vi "Simple Network Streams - Target.vi"() -> ()   [LabVIEW 2015]
doc: "Demonstrates how to use Network Streams to pass data and commands between two running VIs. This VI passes data to the host VI, based on the frequency specified by the host VI."
uses:
  Control 1.ctl
  <vilib>/Platform/TimedLoop/XDataNode/timing_clust.ctl
  <vilib>/Platform/TimedLoop/XDataNode/nitl_modes.ctl
  <vilib>/Platform/TimedLoop/XDataNode/wakeup.ctl
  <vilib>/platform/TimedLoop/XDataNode/XDataNode.xnode
  <vilib>/ErrorRing/Error Ring.xnode
  <vilib>/Platform/TimedLoop/XDataNode/XDNodeRunTimeDep.lvlib
panel:
  out "Time":u32
  out "Counter":i32
  out "output cluster":T1
  in  "Stop":bool
  # "Overview: Demonstrates how to use Network Streams to pass data and commands between two running VIs.\nRequirements: Windows\nInstructions:\n1. Run this VI.\n2. Open Simple Network Streams - Host.vi and follow the instructions on its front panel."
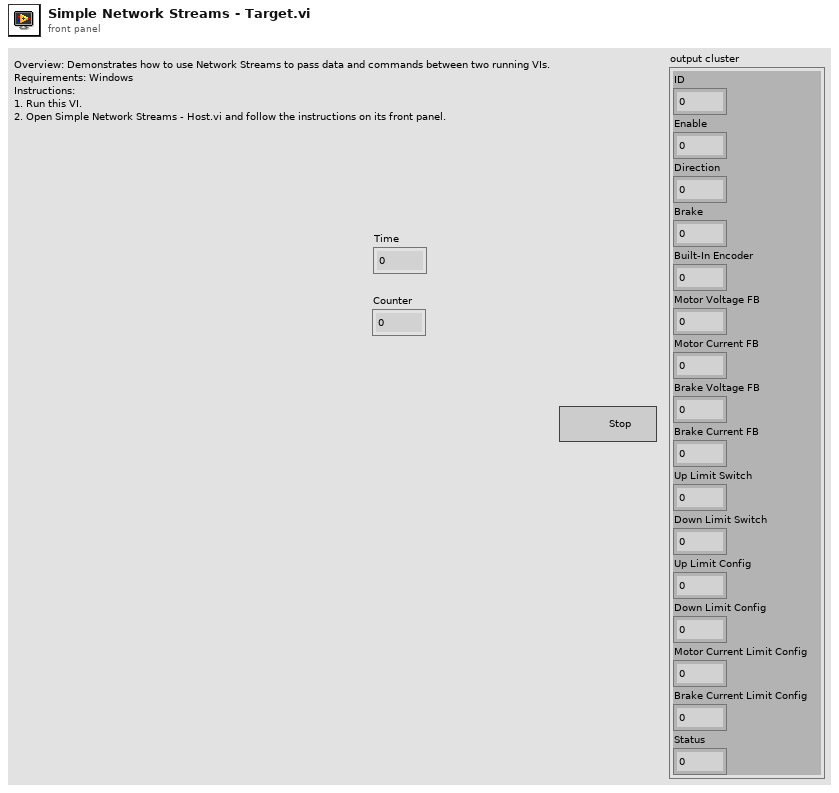
[diagram p1: front panel]
types:
  T1 = typedef "Control 1.ctl" = cluster{"ID":dbl, "Enable":dbl, "Direction":dbl, "Brake":dbl, "Built-In Encoder":dbl, "Motor Voltage FB":dbl, "Motor Current FB":dbl, "Brake Voltage FB":dbl, "Brake Current FB":dbl, "Up Limit Switch":dbl, "Down Limit Switch":dbl, "Up Limit Config":dbl, "Down Limit Config":dbl, "Motor Current Limit Config":dbl, "Brake Current Limit Config":dbl, "Status":dbl}
  T2 = cluster{"ID":dbl, "Enable":dbl, "Direction":dbl, "Brake":dbl, "Built-In Encoder":dbl, "Motor Voltage FB":dbl, "Motor Current FB":dbl, "Brake Voltage FB":dbl, "Brake Current FB":dbl, "Up Limit Switch":dbl, "Down Limit Switch":dbl, "Up Limit Config":dbl, "Down Limit Config":dbl, "Motor Current Limit Config":dbl, "Brake Current Limit Config":dbl, "Status":dbl}
  T3 = typedef "XDNodeRunTimeDep.lvlib/timing_clust.ctl" = cluster{"Expected End [f-1]":u64, "Actual End [f-1]":u64, "Finished Late? [f-1]":bool, "Expected End [i-1]":u64, "Actual End [i-1]":u64, "Finished Late? [i-1]":bool, "Expected Start [i]":u64, "Actual Start [i]":u64, "Expected Start [f]":u64, "Actual Start [f]":u64, "Source Name":string, "Structure Name":string, "Period":i64, "Deadline":i64, "Offset":i64, "Start":i64, "Priority":i32, "Timeout":i32, "Mode":T4, "Wakeup Reason":T5, "Error":errorcluster, "Source Type":string, "Secondary Source Type":string, "Global End Time":u64, "Global Start Time":u64, "Frame Duration":u64, "Iteration Duration":u64, "Assigned CPU":i32, "I/O Scan Engine Mode":u32}
  T4 = typedef "XDNodeRunTimeDep.lvlib/nitl_modes.ctl" = enum32{"No Change", "Process missed periods, maintain original phase", "Discard missed periods, maintain original phase", "Process missed periods, ignore original phase", "Discard missed periods, ignore original phase"}
  T5 = typedef "XDNodeRunTimeDep.lvlib/wakeup.ctl" = enum32{"Normal", "Aborted", "Asynchronous wakeup", "Timing source error", "Timed loop error", "Timeout"}
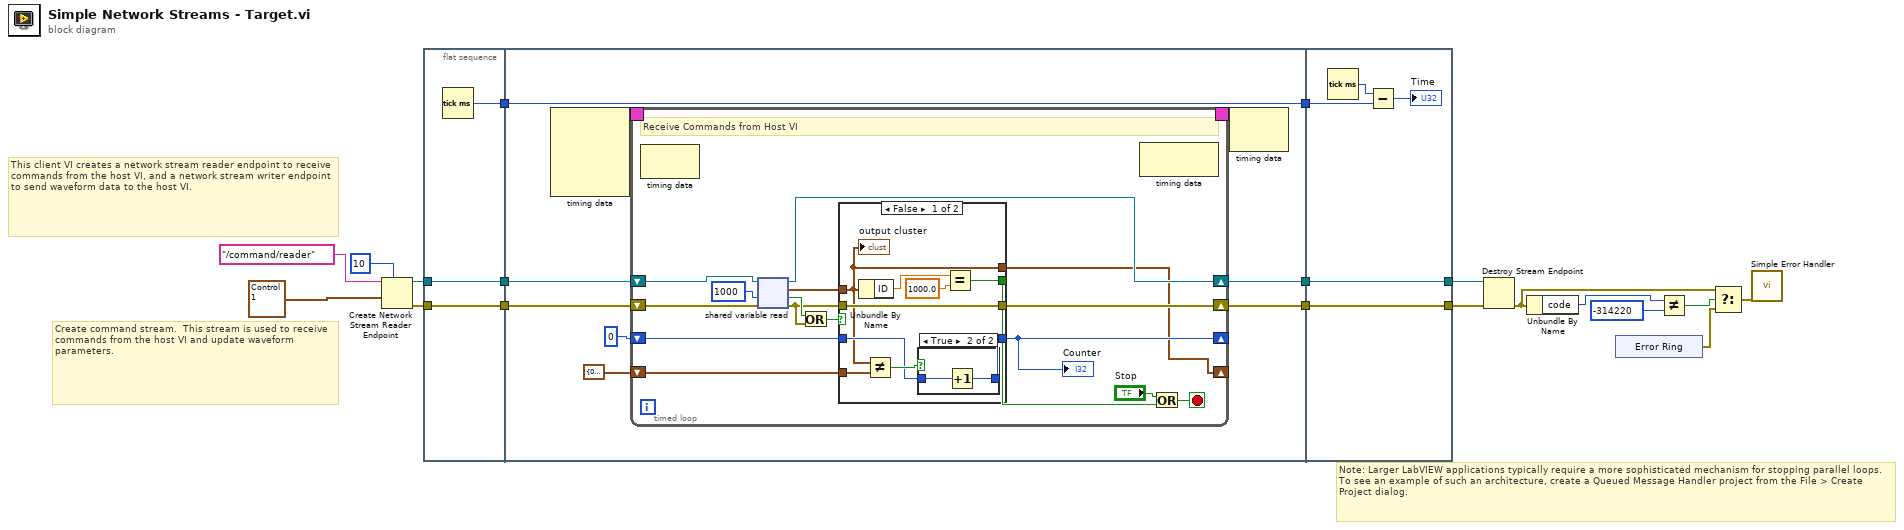
[diagram p0: block diagram]
diagram:
  # "This client VI creates a network stream reader endpoint to receive commands from the host VI, and a network stream writer endpoint to send waveform data to the host VI."
  # "Note: Larger LabVIEW applications typically require a more sophisticated mechanism for stopping parallel loops. To see an example of such an architecture, create a Queued Message Handler project from the File > Create Project dialog."
  # "Create command stream.  This stream is used to receive commands from the host VI and update waveform parameters."
  n1 = Create Network Stream Reader Endpoint(7:10 ("reader buffer size"), 9:T1 {"ID"=0.0, "Enable"=0.0, "Direction"=0.0, "Brake"=0.0, "Built-In Encoder"=0.0, "Motor Voltage FB"=0.0, "Motor Current FB"=0.0, "Brake Voltage FB"=0.0, "Brake Current FB"=0.0, "Up Limit Switch"=0.0, "Down Limit Switch"=0.0, "Up Limit Config"=0.0, "Down Limit Config"=0.0, "Motor Current Limit Config"=0.0, "Brake Current Limit Config"=0.0, "Status"=0.0} ("output cluster"), 11:"/command/reader" ("reader url")) -> (0:w17:errorcluster, 3:w18:refnum<k21>)  [unwired: 4 in]
  n2 = flat-sequence {
    tunnel: w17 -> [w21]
    tunnel: w18 -> [w22]
    tunnel: [w22] -> w6
    tunnel: [w21] -> w5
    tunnel: [w20] -> w1
    tunnel: w6 -> [w31]
    tunnel: w5 -> [w30]
    tunnel: [w29] -> w4
    tunnel: [w28] -> w3
    tunnel: [w26] -> w2
    tunnel: w1 -> [w26]
    tunnel: [w70] -> w15
    tunnel: [w71] -> w16
    tunnel: w4 -> [w71]
    tunnel: w3 -> [w70]
    tunnel: w2 -> [w68]
    frame #0 {
      n3 = Tick Count (ms)() -> (millisecond timer value=w20:u32)
    }
    frame #1 {
      n4 = node-c288() -> (w25:T3)  [unwired: 4 in]
      n5 = timed-loop "Host->Target Command Reader" {
        shift-right: [w43] -> w29
        shift-left: w30 -> [w47]
        shift-right: [w45] -> w28
        shift-left: w31 -> [w46]
        shift-right: [w34] -> _
        shift-left: 0 -> [w35]
        timing: w25 -> [_]
        timing-out: [_] -> w24
        shift-right: [w32] -> _
        shift-left: T2 {"ID"=0.0, "Enable"=0.0, "Direction"=0.0, "Brake"=0.0, "Built-In Encoder"=0.0, "Motor Voltage FB"=0.0, "Motor Current FB"=0.0, "Brake Voltage FB"=0.0, "Brake Current FB"=0.0, "Up Limit Switch"=0.0, "Down Limit Switch"=0.0, "Up Limit Config"=0.0, "Down Limit Config"=0.0, "Motor Current Limit Config"=0.0, "Brake Current Limit Config"=0.0, "Status"=0.0} ("MirrorCoverMotor") -> [w33]
        stop <- w39 stop-if-true
        # "Receive Commands from Host VI"
        n6 = node-c288() -> ()  [unwired: 1 in, 1 out]
        n7 = shared-variable-read(w46, w47, 1000 ("timeout ms")) -> (w45:refnum<k21>, w36:errorcluster, w38:bool, w41:T1)
        n8 = Or(x=w38, y=w36) -> (x .or. y?=w37:bool)
        n9 = case shown="False" w37 {
          tunnel: w36 -> [w55 w64]
          tunnel: [w55 w64] -> w43
          tunnel: w41 -> [w50 w62]
          tunnel: [w56 _] -> w40
          tunnel: w35 -> [w52 w63]
          tunnel: [w51 w63] -> w34
          tunnel: w33 -> [w54 _]
          tunnel: [w50 w62] -> w32
          frame False {
            n10 = Unbundle By Name(w50) -> ("ID"=w58:dbl)
            n11 = Not Equal?(x=w50, y=w54) -> (x != y?=w53:bool)
            n12 = case shown="True" w53 {
              tunnel: w52 -> [w59 w61]
              tunnel: [w59 w60] -> w51
              frame False {
              }
              frame True {
                n13 = Increment(x=w61) -> (x+1=w60:i32)
              }
            }
            n14 = Equal?(x=w58, y=1000.0) -> (x = y?=w56:bool)
            "output cluster" <- w50
          }
          frame True {
          }
        }
        "Counter" <- w34
        n15 = node-c288() -> ()  [unwired: 1 in, 1 out]
        n16 = Or(x="Stop", y=w40) -> (x .or. y?=w39:bool)
      }
      n17 = node-c288(w24) -> ()  [unwired: 1 out]
    }
    frame #2 {
      n18 = Tick Count (ms)() -> (millisecond timer value=w69:u32)
      n19 = Subtract(x=w69, y=w68) -> (x-y=→"Time":u32)
    }
  }
  n20 = Destroy Stream Endpoint(8:w16, 11:w15) -> (0:w9:errorcluster)
  n21 = Unbundle By Name(w9) -> ("code"=w10:i32)
  n22 = xnode "Error Ring"() -> ("error out"=w13:errorcluster)
  n23 = Not Equal?(x=w10, y=-314220) -> (x != y?=w12:bool)
  n24 = Select(t=w9, s=w12, f=w13) -> (s? t:f=w8:errorcluster)
  n25 = call <vilib>:"Simple Error Handler.vi"("error in (no error)"=w8) -> ()  [unwired: 4 in, 5 out]
